vi "1820 State History.vi"(10 "initialize?":bool, 11 "Current State in":string) -> (2 "Current State out":string, 3 "delimited string":string)   [LabVIEW 2019, in "Instrument.Oxford1820.lvclass"]
uses:
  Instrument.Oxford1820.lvclass
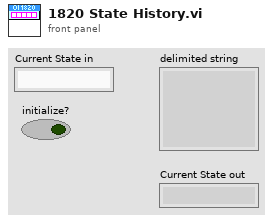
[diagram p1: front panel]
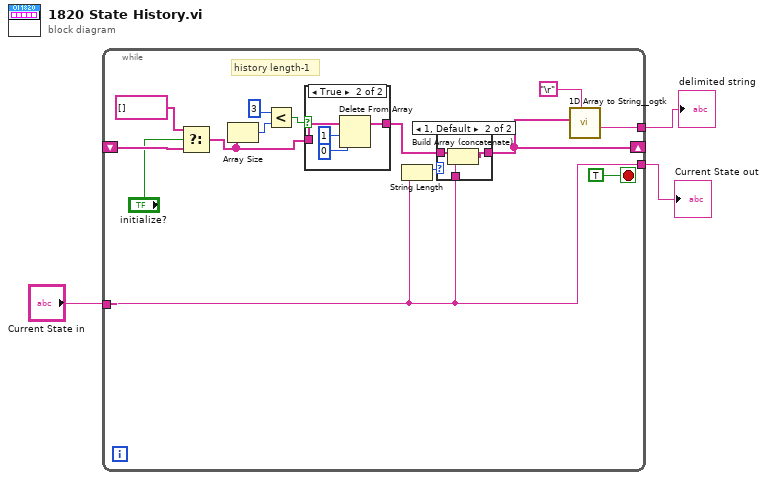
[diagram p0: block diagram]
diagram:
  n1 = while {
    tunnel: [w17] -> w2
    tunnel: "Current State in" -> [w9]
    tunnel: [w9] -> w3
    shift-right: [w8] -> _
    shift-left: _ -> [w7]
    stop <- TRUE stop-if-true
    # "history length-1"
    n2 = Select(t=string[] [], s="initialize?", f=w7) -> (s? t:f=w6:string[])
    n3 = Array Size(array=w6) -> (size(s)=w14:i32)
    n4 = Less?(x=3 ("length"), y=w14) -> (x < y?=w16:bool)
    n5 = case shown="True" w16 {
      tunnel: w6 -> [w22 w23]
      tunnel: [w22 w25] -> w15
      frame False {
      }
      frame True {
        n6 = Delete From Array(array=w23, length=1, index=0) -> (array with subset deleted=w25:string[])  [unwired: 1 out]
      }
    }
    n7 = String Length(string=w9) -> (length=w13:i32)
    n8 = case shown="1, Default" w13 {
      tunnel: w15 -> [w18 w21]
      tunnel: [w18 w20] -> w8
      tunnel: w9 -> [_ w19]
      frame 0 {
      }
      frame 1, Default {
        n9 = Build Array (concatenate)(w21, w19) -> (w20:string[])
      }
    }
    n10 = call <userlib>:"1D Array to String__ogtk.vi"("delimiter (Tab)"="\r", "Array of Strings"=w8) -> ("delimited string"=w17:string)  [unwired: 9 in]
  }
  "Current State out" <- w3
  "delimited string" <- w2
